vi "Graph Ramp.vi"(0 "Start (Volts)":dbl format="%.2f", 5 "End (volts)":dbl format="%.2f", 7 "Voltage Increment":dbl format="%.2f", 9 "Dwell (sec)":dbl format="%.5f") -> (6 "Voltage vs Time":cluster{dbl[], dbl[]}(graph))   [LabVIEW 2013]
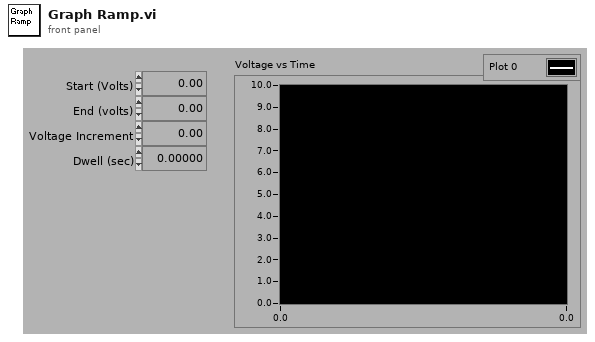
[diagram p1: front panel]
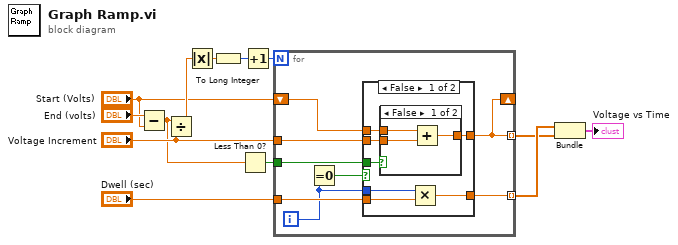
[diagram p0: block diagram]
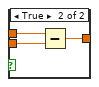
[diagram p2: hidden frame]
diagram:
  n1 = Subtract(x="End (volts)", y="Start (Volts)") -> (x-y=w5:dbl)
  n2 = Divide(x=w5, y="Voltage Increment") -> (x/y=w9:dbl)
  n3 = Absolute Value(x=w9) -> (abs(x)=w13:dbl)
  n4 = To Long Integer(number=w13) -> (32bit integer=w12:i32)
  n5 = Less Than 0?(x=w5) -> (x < 0?=w6:bool)
  n6 = Increment(x=w12) -> (x+1=w11:i32)
  n7 = for {
    N: w11 -> [_]
    shift-right: [w19] -> _
    shift-left: "Start (Volts)" -> [w18]
    tunnel: "Voltage Increment" -> [w21]
    tunnel: w6 -> [w20]
    tunnel: [w19] -> w1 mode=indexing
    tunnel: "Dwell (sec)" -> [w15]
    tunnel: [w16] -> w3 mode=indexing
    i -> [w14]
    n8 = Equal To 0?(x=w14) -> (x = 0?=w17:bool)
    n9 = case shown="False" w17 {
      tunnel: w21 -> [w27 _]
      tunnel: w20 -> [w26 _]
      tunnel: [w25 w36] -> w19
      tunnel: w18 -> [w28 w36]
      tunnel: w14 -> [w24 w35]
      tunnel: [w22 w35] -> w16
      tunnel: w15 -> [w23 _]
      frame False {
        n10 = case shown="False" w26 {
          tunnel: w28 -> [w30 w34]
          tunnel: w27 -> [w29 w33]
          tunnel: [w31 w32] -> w25
          frame False {
            n11 = Add(x=w30, y=w29) -> (x+y=w31:dbl)
          }
          frame True {
            n12 = Subtract(x=w34, y=w33) -> (x-y=w32:dbl)
          }
        }
        n13 = Multiply(x=w24, y=w23) -> (x*y=w22:dbl)
      }
      frame True {
      }
    }
  }
  n14 = Bundle(w3, w1) -> (→"Voltage vs Time":cluster{dbl[], dbl[]})  [unwired: 1 out]
